vi "Switch-DMM Initialization VI.vi"(8 "error in (no error)":errorcluster, 10 "Custom XML":string, 11 "Device Item Ref in":T1 format="%.0x") -> (0 "error out":errorcluster, 3 "Device Item Ref out":T1 format="%.0x")   [LabVIEW 2011, in "Switch-DMM Custom Device.lvlib"]
uses:
  Switch-DMM Custom Device.lvlib
  <vilib>/NI Veristand/Custom Device API/Custom Device Item Ref.ctl
  <vilib>/NI Veristand/Custom Device API/Custom Device Channel.ctl
  <vilib>/NI Veristand/Custom Device API/Custom Device Channel Type.ctl
  Controls/Globals.vi
  <vilib>/NI Veristand/Custom Device API/Set Item Property (String).vi
  <vilib>/NI Veristand/Custom Device API/Set Item Property (U16).vi
  <vilib>/NI Veristand/Custom Device API/Set Item Property (Double).vi
  <vilib>/NI Veristand/Custom Device API/Set Item Property (I32).vi
  <vilib>/NI Veristand/Custom Device API/Set Item Property (Boolean).vi
  <vilib>/NI Veristand/Custom Device API/Custom Device API.lvlib
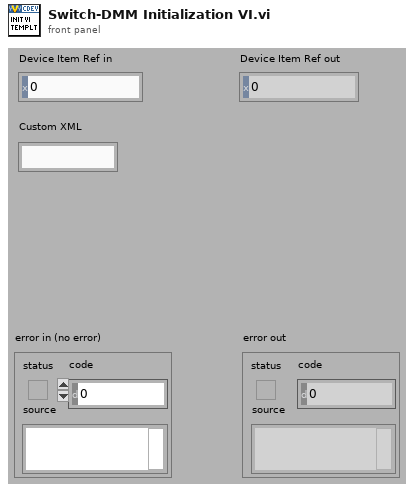
[diagram p1: front panel]
types:
  T1 = typedef "Custom Device API.lvlib/Custom Device Item Ref.ctl" = u64
  T2 = typedef "Custom Device API.lvlib/Custom Device Channel.ctl" = cluster{"Type":T3, "Units":string, "Default Value":dbl, "Faultable":bool, "Scalable":bool}
  T3 = typedef "Custom Device API.lvlib/Custom Device Channel Type.ctl" = enum16{"Input", "Output"}
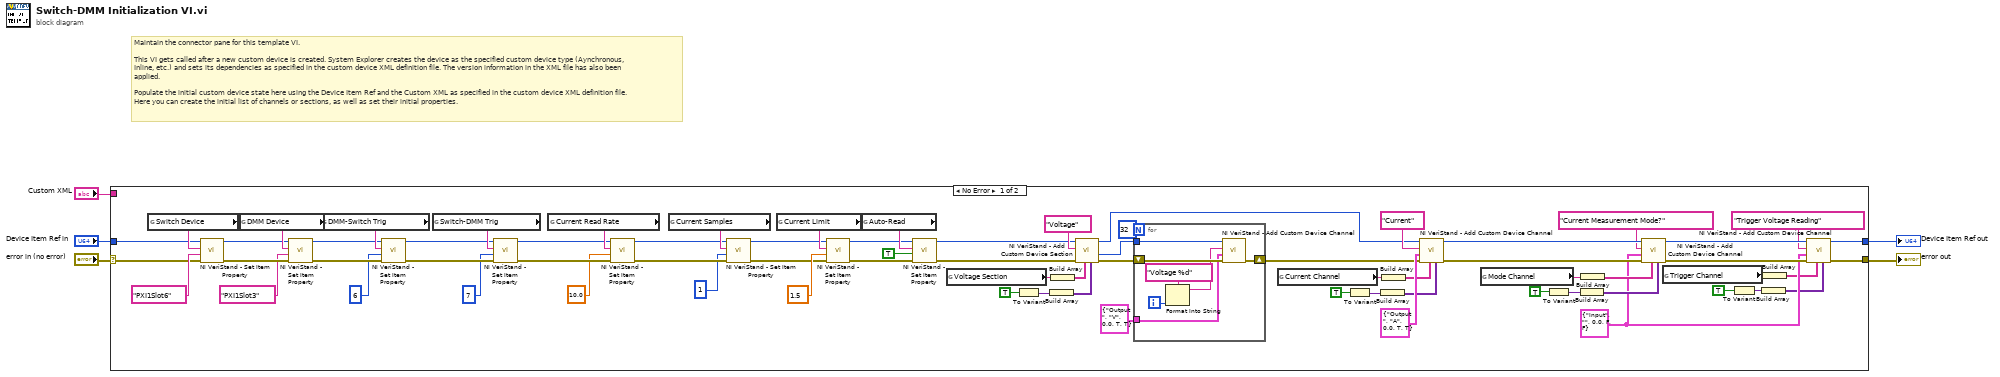
[diagram p0: block diagram]
diagram:
  # "Maintain the connector pane for this template VI.\n\nThis VI gets called after a new custom device is created. System Explorer creates the device as the specified custom device type (Aynchronous, Inline, etc.) and sets its dependencies as specified in the custom device XML definition file. The version information in the XML file has also been applied.\n\nPopulate the initial custom device state here using the Device Item Ref and the Custom XML as specified in the custom device XML definition file. Here you can create the initial list of channels or sections, as well as set their initial properties."
  n1 = case shown="No Error" "error in (no error)" {
    selector: "error in (no error)" -> [w50 w86]
    tunnel: [w18 w86] -> w5
    tunnel: [w19 w85] -> w3
    tunnel: "Device Item Ref in" -> [w51 w85]
    tunnel: "Custom XML" -> [_ _]
    frame No Error {
      w25 = T2 {"Type"=enum."Input", "Units"="", "Default Value"=0.0, "Faultable"=FALSE, "Scalable"=FALSE} ("Channel")
      n2 = global read "Globals.vi" "Switch Device"() -> (w71:string)
      n3 = call-poly <vilib>:"NI VeriStand - Set Item Property.vi"("error in (no error)"=w50, "Value"="PXI1Slot6", "Property Name"=w71, "Item Ref in"=w51) -> ("error out"=w68:errorcluster, "Item Ref out"=w69:T1)  [unwired: 5 in, 1 out]
      n4 = global read "Globals.vi" "DMM Device"() -> (w70:string)
      n5 = call-poly <vilib>:"NI VeriStand - Set Item Property.vi"("error in (no error)"=w68, "Value"="PXI1Slot3", "Property Name"=w70, "Item Ref in"=w69) -> ("error out"=w65:errorcluster, "Item Ref out"=w66:T1)  [unwired: 5 in, 1 out]
      n6 = global read "Globals.vi" "DMM-Switch Trig"() -> (w67:string)
      n7 = call-poly <vilib>:"NI VeriStand - Set Item Property.vi"("error in (no error)"=w65, "Value"=u16 6, "Property Name"=w67, "Item Ref in"=w66) -> ("error out"=w62:errorcluster, "Item Ref out"=w63:T1)  [unwired: 5 in, 1 out]
      n8 = global read "Globals.vi" "Switch-DMM Trig"() -> (w64:string)
      n9 = call-poly <vilib>:"NI VeriStand - Set Item Property.vi"("error in (no error)"=w62, "Value"=u16 7, "Property Name"=w64, "Item Ref in"=w63) -> ("error out"=w59:errorcluster, "Item Ref out"=w60:T1)  [unwired: 5 in, 1 out]
      n10 = global read "Globals.vi" "Current Read Rate"() -> (w61:string)
      n11 = call-poly <vilib>:"NI VeriStand - Set Item Property.vi"("error in (no error)"=w59, "Value"=10.0, "Property Name"=w61, "Item Ref in"=w60) -> ("error out"=w9:errorcluster, "Item Ref out"=w10:T1)  [unwired: 5 in, 1 out]
      n12 = global read "Globals.vi" "Current Samples"() -> (w11:string)
      n13 = call-poly <vilib>:"NI VeriStand - Set Item Property.vi"("error in (no error)"=w9, "Value"=1, "Property Name"=w11, "Item Ref in"=w10) -> ("error out"=w6:errorcluster, "Item Ref out"=w7:T1)  [unwired: 5 in, 1 out]
      n14 = global read "Globals.vi" "Current Limit"() -> (w58:string)
      n15 = call-poly <vilib>:"NI VeriStand - Set Item Property.vi"("error in (no error)"=w6, "Value"=1.5, "Property Name"=w58, "Item Ref in"=w7) -> ("error out"=w15:errorcluster, "Item Ref out"=w16:T1)  [unwired: 5 in, 1 out]
      n16 = global read "Globals.vi" "Auto-Read"() -> (w17:string)
      n17 = call-poly <vilib>:"NI VeriStand - Set Item Property.vi"("error in (no error)"=w15, "Value"=TRUE, "Property Name"=w17, "Item Ref in"=w16) -> ("error out"=w12:errorcluster, "Item Ref out"=w13:T1)  [unwired: 5 in, 1 out]
      n18 = global read "Globals.vi" "Voltage Section"() -> (w76:string)
      n19 = To Variant(anything=TRUE) -> (Variant=w73:variant)
      n20 = Build Array(w73) -> (w72:variant[])
      n21 = Build Array(w76) -> (w75:string[])
      n22 = call <vilib>:"NI VeriStand - Add Custom Device Section.vi"("Property Values"=w72, "Property names"=w75, "error in (no error)"=w12, "Section Name"="Voltage", "Parent Ref in"=w13) -> ("error out"=w45:errorcluster, "Section Ptr"=w44:T1, "Parent Ref out"=w39:T1)  [unwired: 3 in, 1 out]
      n23 = for {
        N: 32 -> [_]
        shift-right: [w83] -> w37
        shift-left: w45 -> [w84]
        tunnel: w44 -> [w82]
        tunnel: T2 {"Type"=enum."Output", "Units"="V", "Default Value"=0.0, "Faultable"=TRUE, "Scalable"=TRUE} ("Channel") -> [w79]
        i -> [w81]
        n24 = Format Into String(format string="Voltage %d", w81) -> (resulting string=w78:string)  [unwired: 2 in, 1 out]
        n25 = call <vilib>:"NI VeriStand - Add Custom Device Channel.vi"("error in (no error)"=w84, "Channel"=w79, "Channel Name"=w78, "Parent Ref in"=w82) -> ("error out"=w83:errorcluster)  [unwired: 4 in, 3 out]
      }
      n26 = global read "Globals.vi" "Current Channel"() -> (w47:string)
      n27 = To Variant(anything=TRUE) -> (Variant=w49:variant)
      n28 = Build Array(w49) -> (w36:variant[])
      n29 = Build Array(w47) -> (w35:string[])
      n30 = call <vilib>:"NI VeriStand - Add Custom Device Channel.vi"("Property Values"=w36, "Property names"=w35, "error in (no error)"=w37, "Channel"=T2 {"Type"=enum."Output", "Units"="A", "Default Value"=0.0, "Faultable"=TRUE, "Scalable"=TRUE}, "Channel Name"="Current" ("Section Name"), "Parent Ref in"=w39) -> ("error out"=w40:errorcluster, "Parent Ref out"=w38:T1)  [unwired: 2 in, 2 out]
      n31 = global read "Globals.vi" "Mode Channel"() -> (w33:string)
      n32 = To Variant(anything=TRUE) -> (Variant=w31:variant)
      n33 = Build Array(w31) -> (w29:variant[])
      n34 = Build Array(w33) -> (w30:string[])
      n35 = call <vilib>:"NI VeriStand - Add Custom Device Channel.vi"("Property Values"=w29, "Property names"=w30, "error in (no error)"=w40, "Channel"=w25, "Channel Name"="Current Measurement Mode?" ("Section Name"), "Parent Ref in"=w38) -> ("error out"=w27:errorcluster, "Parent Ref out"=w28:T1)  [unwired: 2 in, 2 out]
      n36 = global read "Globals.vi" "Trigger Channel"() -> (w22:string)
      n37 = To Variant(anything=TRUE) -> (Variant=w24:variant)
      n38 = Build Array(w24) -> (w20:variant[])
      n39 = Build Array(w22) -> (w21:string[])
      n40 = call <vilib>:"NI VeriStand - Add Custom Device Channel.vi"("Property Values"=w20, "Property names"=w21, "error in (no error)"=w27, "Channel"=w25, "Channel Name"="Trigger Voltage Reading" ("Section Name"), "Parent Ref in"=w28) -> ("error out"=w18:errorcluster, "Parent Ref out"=w19:T1)  [unwired: 2 in, 2 out]
    }
    frame Error {
    }
  }
  "error out" <- w5
  "Device Item Ref out" <- w3
